vi "Calculate Quaternion From Rotation Matrix.vi"(0 "Rotation Matrix":T1) -> (1 "appended array":dbl[](array[numeric]), 2 "|q|":dbl)   [LabVIEW 2021, in "IMU Processing.lvlib"]
uses:
  IMU Processing.lvlib
  <vilib>/Analysis/Matrix/Datatypes/RealMatrix.ctl
  <vilib>/Analysis/_algsub.llb/Real Matrix Norm.vi
  <vilib>/Analysis/Matrix/Numeric/Conversions/Array To Matrix - RA.vi
  <vilib>/Analysis/NI_AALPro.lvlib
  <vilib>/Analysis/Matrix/NI_Matrix.lvlib
panel:
  out "qz":dbl
  out "qy":dbl
  out "qw":dbl
  out "qx":dbl
  out "gcode":dbl
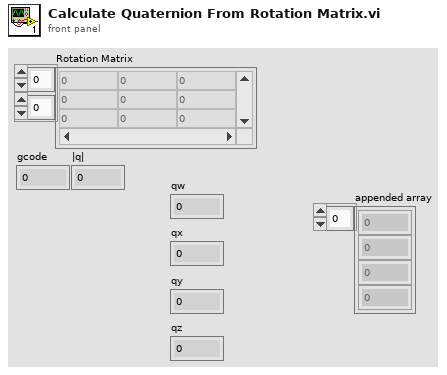
[diagram p1: front panel]
types:
  T1 = typedef "NI_Matrix.lvlib/RealMatrix.ctl" = dbl[][]
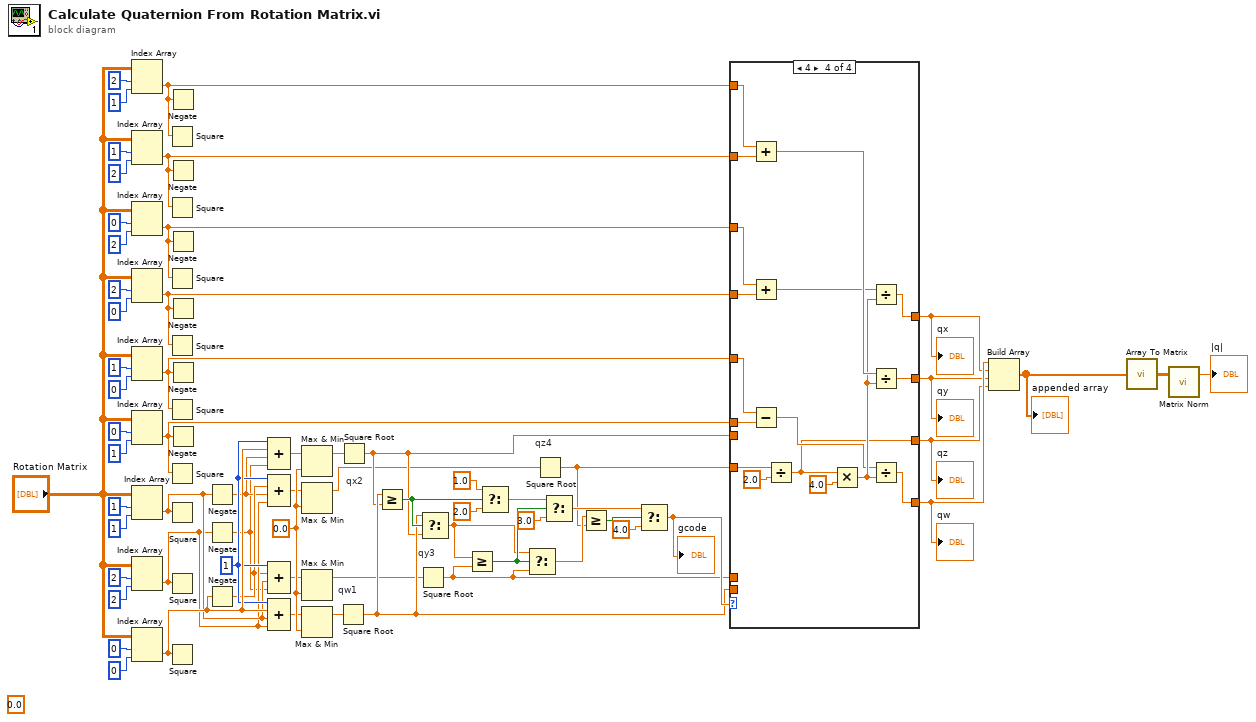
[diagram p0: block diagram]
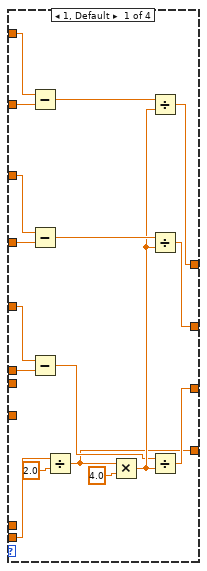
[diagram p2: hidden frame]
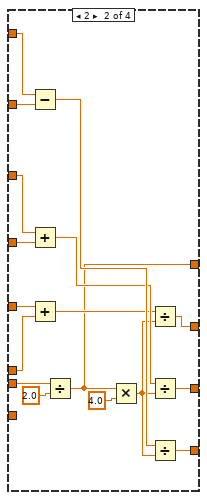
[diagram p3: hidden frame]
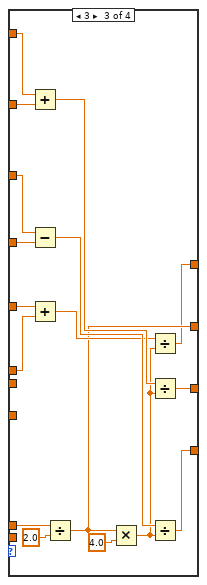
[diagram p4: hidden frame]
diagram:
  (unwired) 0.0 ("y")
  w7 = 0.0 ("y")
  w44 = 1
  n1 = Index Array(array="Rotation Matrix", index (row)=2, index (col)=1) -> (element=w26:dbl)
  n2 = Index Array(array="Rotation Matrix", index (row)=1, index (col)=2) -> (element=w25:dbl)
  n3 = Index Array(array="Rotation Matrix", index (row)=0, index (col)=2) -> (element=w24:dbl)
  n4 = Index Array(array="Rotation Matrix", index (row)=2, index (col)=0) -> (element=w23:dbl)
  n5 = Index Array(array="Rotation Matrix", index (row)=1, index (col)=0) -> (element=w22:dbl)
  n6 = Index Array(array="Rotation Matrix", index (row)=0, index (col)=1) -> (element=w21:dbl)
  n7 = Index Array(array="Rotation Matrix", index (row)=1, index (col)=1) -> (element=w43:dbl)
  n8 = Index Array(array="Rotation Matrix", index (row)=2, index (col)=2) -> (element=w42:dbl)
  n9 = Index Array(array="Rotation Matrix", index (row)=0, index (col)=0) -> (element=w45:dbl)
  n10 = Square(x=w26) -> ()  [unwired: 1 out]
  n11 = Square(x=w25) -> ()  [unwired: 1 out]
  n12 = Square(x=w24) -> ()  [unwired: 1 out]
  n13 = Square(x=w23) -> ()  [unwired: 1 out]
  n14 = Square(x=w22) -> ()  [unwired: 1 out]
  n15 = Square(x=w21) -> ()  [unwired: 1 out]
  n16 = Square(x=w43) -> ()  [unwired: 1 out]
  n17 = Square(x=w42) -> ()  [unwired: 1 out]
  n18 = Square(x=w45) -> ()  [unwired: 1 out]
  n19 = Negate(x=w26) -> ()  [unwired: 1 out]
  n20 = Negate(x=w25) -> ()  [unwired: 1 out]
  n21 = Negate(x=w24) -> ()  [unwired: 1 out]
  n22 = Negate(x=w23) -> ()  [unwired: 1 out]
  n23 = Negate(x=w22) -> ()  [unwired: 1 out]
  n24 = Negate(x=w21) -> ()  [unwired: 1 out]
  n25 = Negate(x=w43) -> (-x=w40:dbl)
  n26 = Negate(x=w42) -> (-x=w39:dbl)
  n27 = Negate(x=w45) -> (-x=w41:dbl)
  n28 = Compound Arithmetic op=ADD(w44, w45, w40, w39) -> (w9:dbl)
  n29 = Compound Arithmetic op=ADD(w44, w41, w40, w42) -> (w6:dbl)
  n30 = Compound Arithmetic op=ADD(w44, w41, w43, w39) -> (w5:dbl)
  n31 = Compound Arithmetic op=ADD(w44, w45, w43, w42) -> (w4:dbl)
  n32 = Max & Min(x=w9, y=w7) -> (max(x,y)=w8:dbl)  [unwired: 1 out]
  n33 = Max & Min(x=w6, y=w7) -> (max(x,y)=w1:dbl)  [unwired: 1 out]
  n34 = Max & Min(x=w5, y=w7) -> (max(x,y)=w2:dbl)  [unwired: 1 out]
  n35 = Max & Min(x=w4, y=w7) -> (max(x,y)=w3:dbl)  [unwired: 1 out]
  n36 = Square Root "qw1"(x=w3) -> (sqrt(x)=w20:dbl)
  n37 = Square Root "qx2"(x=w8) -> (sqrt(x)=w19:dbl)
  n38 = Greater Or Equal?(x=w20, y=w19) -> (x >= y?=w36:bool)
  n39 = Square Root "qy3"(x=w2) -> (sqrt(x)=w18:dbl)
  n40 = Select(t=w20, s=w36, f=w19) -> (s? t:f=w32:dbl)
  n41 = Greater Or Equal?(x=w32, y=w18) -> (x >= y?=w33:bool)
  n42 = Select(t=1.0, s=w36, f=2.0) -> (s? t:f=w35:dbl)
  n43 = Select(t=w32, s=w33, f=w18) -> (s? t:f=w29:dbl)
  n44 = Square Root "qz4"(x=w1) -> (sqrt(x)=w17:dbl)
  n45 = Select(t=w35, s=w33, f=3.0) -> (s? t:f=w28:dbl)
  n46 = Greater Or Equal?(x=w29, y=w17) -> (x >= y?=w30:bool)
  n47 = Select(t=w28, s=w30, f=4.0) -> (s? t:f=w27:dbl)
  "gcode" <- w27
  n48 = case shown="4" w27 {
    tunnel: w26 -> [w81 w98 w115 w132]
    tunnel: w25 -> [w80 w97 w114 w131]
    tunnel: [w66 w84 w100 w118] -> w16
    tunnel: [w77 w85 w101 w117] -> w15
    tunnel: w24 -> [w73 w91 w108 w125]
    tunnel: w23 -> [w72 w90 w107 w124]
    tunnel: w22 -> [w71 w89 w106 w123]
    tunnel: w21 -> [w70 w88 w105 w122]
    tunnel: [w69 w83 w102 w116] -> w14
    tunnel: [w68 w82 w99 w119] -> w13
    tunnel: w20 -> [w65 _ _ _]
    tunnel: w19 -> [_ w86 _ _]
    tunnel: w18 -> [_ _ w103 _]
    tunnel: w17 -> [_ _ _ w120]
    frame 1, Default {
      n49 = Subtract(x=w81, y=w80) -> (x-y=w78:dbl)
      n50 = Subtract(x=w73, y=w72) -> (x-y=w76:dbl)
      n51 = Subtract(x=w71, y=w70) -> (x-y=w74:dbl)
      n52 = Divide(x=w65, y=2.0) -> (x/y=w66:dbl)
      n53 = Multiply(x=w66, y=4.0) -> (x*y=w75:dbl)
      n54 = Divide(x=w78, y=w75) -> (x/y=w77:dbl)
      n55 = Divide(x=w76, y=w75) -> (x/y=w69:dbl)
      n56 = Divide(x=w74, y=w75) -> (x/y=w68:dbl)
    }
    frame 2 {
      n57 = Subtract(x=w98, y=w97) -> (x-y=w95:dbl)
      n58 = Add(x=w91, y=w90) -> (x+y=w94:dbl)
      n59 = Add(x=w89, y=w88) -> (x+y=w92:dbl)
      n60 = Divide(x=w86, y=2.0) -> (x/y=w85:dbl)
      n61 = Multiply(x=w85, y=4.0) -> (x*y=w93:dbl)
      n62 = Divide(x=w92, y=w93) -> (x/y=w83:dbl)
      n63 = Divide(x=w94, y=w93) -> (x/y=w82:dbl)
      n64 = Divide(x=w95, y=w93) -> (x/y=w84:dbl)
    }
    frame 3 {
      n65 = Add(x=w115, y=w114) -> (x+y=w112:dbl)
      n66 = Subtract(x=w108, y=w107) -> (x-y=w111:dbl)
      n67 = Add(x=w106, y=w105) -> (x+y=w109:dbl)
      n68 = Divide(x=w103, y=2.0) -> (x/y=w102:dbl)
      n69 = Multiply(x=w102, y=4.0) -> (x*y=w110:dbl)
      n70 = Divide(x=w109, y=w110) -> (x/y=w101:dbl)
      n71 = Divide(x=w112, y=w110) -> (x/y=w99:dbl)
      n72 = Divide(x=w111, y=w110) -> (x/y=w100:dbl)
    }
    frame 4 {
      n73 = Add(x=w132, y=w131) -> (x+y=w129:dbl)
      n74 = Add(x=w125, y=w124) -> (x+y=w128:dbl)
      n75 = Subtract(x=w123, y=w122) -> (x-y=w126:dbl)
      n76 = Divide(x=w120, y=2.0) -> (x/y=w119:dbl)
      n77 = Multiply(x=w119, y=4.0) -> (x*y=w127:dbl)
      n78 = Divide(x=w128, y=w127) -> (x/y=w117:dbl)
      n79 = Divide(x=w129, y=w127) -> (x/y=w116:dbl)
      n80 = Divide(x=w126, y=w127) -> (x/y=w118:dbl)
    }
  }
  "qx" <- w15
  "qw" <- w16
  "qy" <- w14
  "qz" <- w13
  n81 = Build Array(w16, w15, w14, w13) -> (w12:dbl[])
  "appended array" <- w12
  n82 = call-poly <vilib>:"Array To Matrix.vi"("Real 1D Array"=w12) -> ("Real Matrix (Column Vector)"=w11:T1)
  n83 = call-poly <vilib>:"Matrix Norm.vi"("Input Matrix"=w11) -> ("norm"=→"|q|":dbl)  [unwired: 1 in, 1 out]
